vi "Read Data Bits.vi"(8 "error in (no error)":errorcluster, 11 "RTU Data Unit in":refnum<class "RTU Data Unit.lvclass">) -> (0 "error out":errorcluster, 2 "data bits":u16=8, 3 "RTU Data Unit out":refnum<class "RTU Data Unit.lvclass">)   [LabVIEW 2012, in "RTU Data Unit.lvclass"]
doc: "Acts as a constant, and provides a way for the serial slave to properly configure the serial interface. 8 bits in this case."
uses:
  RTU Data Unit.lvclass
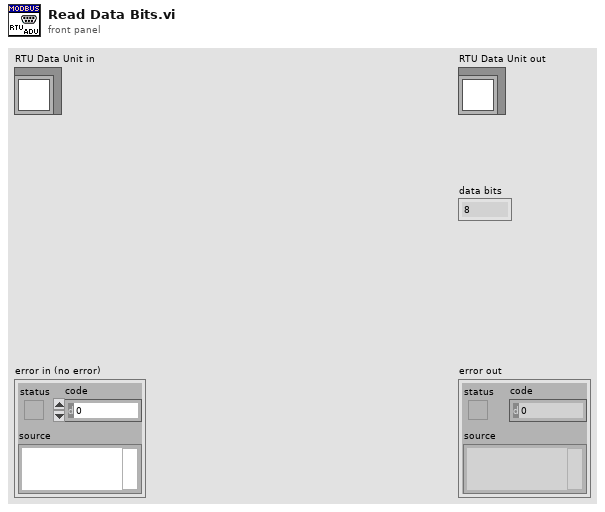
[diagram p1: front panel]
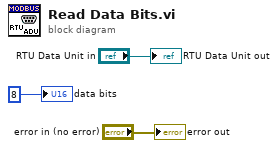
[diagram p0: block diagram]
diagram:
  "error out" <- "error in (no error)"
  "RTU Data Unit out" <- "RTU Data Unit in"
  "data bits" <- u16 8 ("data bits")
